vi "SSP - click.vi"(8 "error in (no error)":errorcluster, 11 "JSON string":string) -> (0 "error out":errorcluster, 3 "value":string)   [LabVIEW 2020, in "ui-testing.lvlib"]
doc: "copyright: Thomas Zilliox©"
uses:
  ui-testing.lvlib
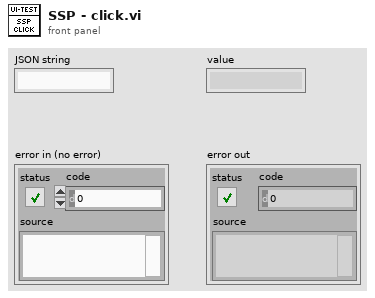
[diagram p1: front panel]
types:
  T1 = cluster{"control":string, "subpanel":string, "subsubpanel":string}
  T2 = cluster{"VI with Focus":refnum<vi>, "SubPanel":refnum<vi>, "SubSubPanel":refnum<vi>, "SubPanel VI":refnum<vi>}
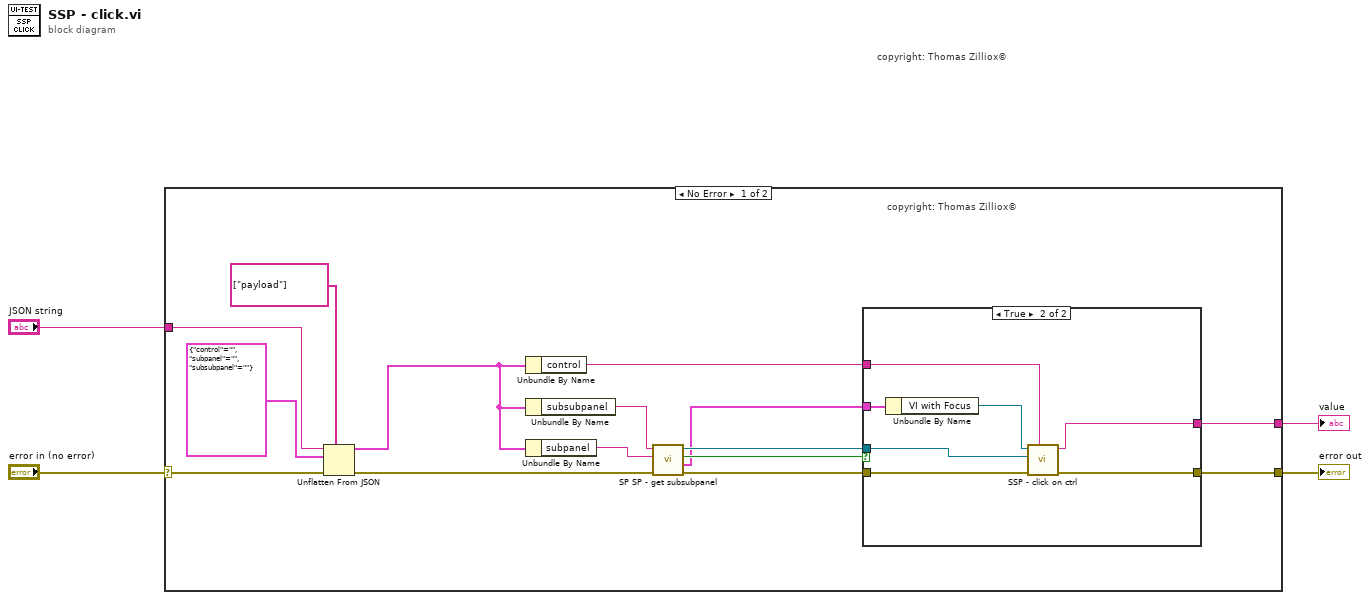
[diagram p0: block diagram]
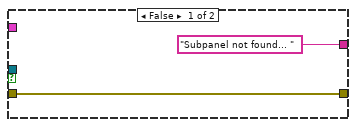
[diagram p2: hidden frame]
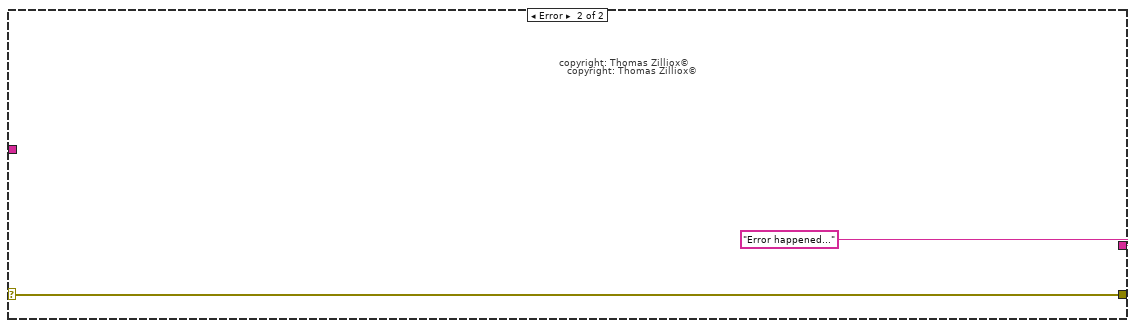
[diagram p3: hidden frame]
diagram:
  # "copyright: Thomas Zilliox©"
  n1 = case shown="No Error" "error in (no error)" {
    selector: "error in (no error)" -> [w15 w30]
    tunnel: "JSON string" -> [w17 _]
    tunnel: [w16 w30] -> w3
    tunnel: [w13 "Error happened..."] -> w1
    frame No Error {
      # "copyright: Thomas Zilliox©"
      n2 = Unflatten From JSON(path=string[] ["payload"], JSON string=w17, type and defaults=T1 {"control"="", "subpanel"="", "subsubpanel"=""}, error in (no error)=w15) -> (value=w12:T1, error out=w18:errorcluster)  [unwired: 3 in]
      n3 = Unbundle By Name(w12) -> ("control"=w7:string)
      n4 = Unbundle By Name(w12) -> ("subsubpanel"=w10:string)
      n5 = Unbundle By Name(w12) -> ("subpanel"=w11:string)
      n6 = call "SP SP - get subsubpanel.vi"("error in (no error)"=w18, "subpanel"=w11, "subsubpanel"=w10) -> ("error out"=w9:errorcluster, "references"=w5:T2, "SubSubPanel found"=w8:bool, "SubSubPanel VI"=w6:refnum<vi>)  [unwired: 5 in]
      n7 = case shown="True" w8 {
        tunnel: [w21 w26] -> w16
        tunnel: w9 -> [w21 w28]
        tunnel: w7 -> [_ w25]
        tunnel: ["Subpanel not found... " ("result string") w27] -> w13
        tunnel: w6 -> [_ w24]
        tunnel: w5 -> [_ w23]
        frame False {
        }
        frame True {
          n8 = Unbundle By Name(w23) -> ("VI with Focus"=w22:refnum<vi>)
          n9 = call "SSP - click on ctrl.vi"("Control Label"=w25, "error in (no error)"=w28, "subVI"=w24, "VI with Focus"=w22) -> ("error out"=w26:errorcluster, "return value"=w27:string)  [unwired: 6 in]
        }
      }
    }
    frame Error {
      # "copyright: Thomas Zilliox©"
      # "copyright: Thomas Zilliox©"
    }
  }
  "error out" <- w3
  "value" <- w1
